vi "COUNTER_INIT.vi"(3 "OptionEdge":dbl=1.0, 4 "error in (no error)":errorcluster, 5 "VISA resource name":refnum<visa-resource-name>) -> (0 "error out":errorcluster, 1 "Edge":u8, 2 "VISA resource Salida":refnum<visa-resource-name>)   [LabVIEW 2011]
panel:
  out "unsigned byte array":u8[](array[numeric])
  out "Read Counter command":u8[](array[numeric])
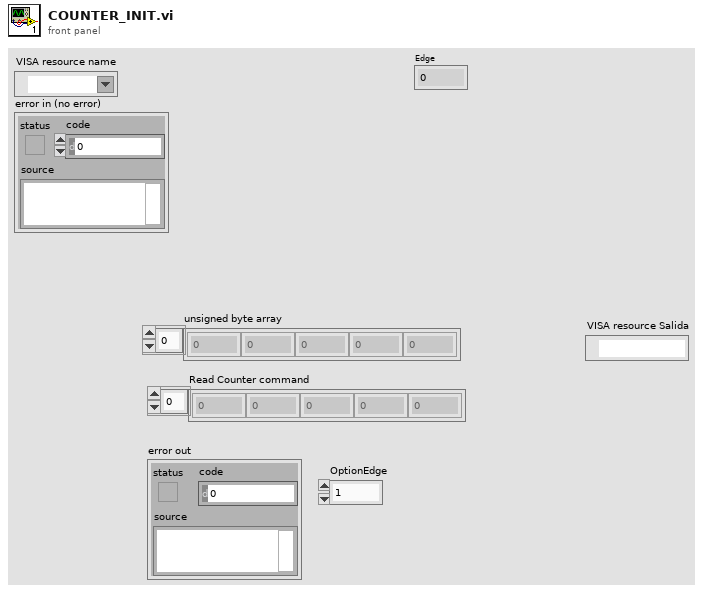
[diagram p1: front panel]
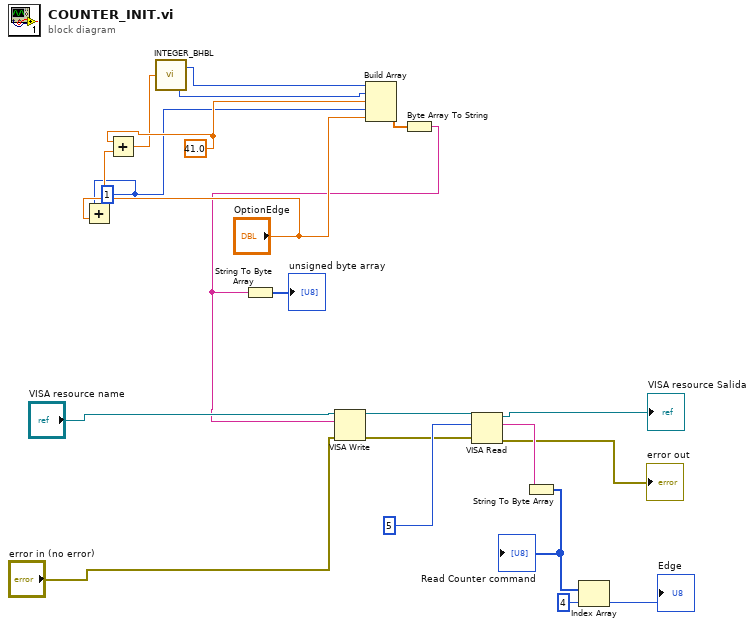
[diagram p0: block diagram]
diagram:
  w1 = 1 ("reset")
  w10 = 41.0 ("element")
  n1 = Add(x=w1, y="OptionEdge") -> (x+y=w11:dbl)
  n2 = Add(x=w10, y=w11) -> (x+y=w9:dbl)
  n3 = call "INTEGER_BHBL.vi"("int16"=w9) -> ("Lvalue"=w7:u8, "HValue"=w8:u8)
  n4 = Build Array(w8, w7, w10, w1, "OptionEdge") -> (w15:dbl[])
  n5 = Byte Array To String(unsigned byte array=w15) -> (string=w6:string)
  n6 = String To Byte Array(string=w6) -> (unsigned byte array=→"unsigned byte array":u8[])
  n7 = VISA Write(VISA resource name="VISA resource name", write buffer=w6, error in (no error)="error in (no error)") -> (VISA resource name out=w16:refnum<visa-resource-name>, error out=w18:errorcluster)  [unwired: 1 out]
  n8 = VISA Read(VISA resource name=w16, byte count=u32 5, error in (no error)=w18) -> (VISA resource name out=→"VISA resource Salida":refnum<visa-resource-name>, read buffer=w20:string, error out=→"error out":errorcluster)  [unwired: 1 out]
  n9 = String To Byte Array(string=w20) -> (unsigned byte array=w4:u8[])
  "Read Counter command" <- w4
  n10 = Index Array(array=w4, index=4) -> (element=→"Edge":u8)
